vi "Refname to String (Actuator).vi"(1 "Actuator Refname":T1) -> (0 "Refnum Name":string)   [LabVIEW 2015, in "Sprocket.lvlib"]
uses:
  lib/Sprocket.lvlib
  Actuators.ctl
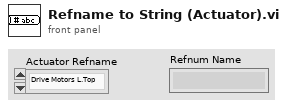
[diagram p1: front panel]
types:
  T1 = typedef "Sprocket.lvlib/Actuators.ctl" = enum16{"Drive Motors L.Top", "Drive Motors R.Top", "Drive Motors L.Bot", "Drive Motors R.Bot", "Collector Motor"}
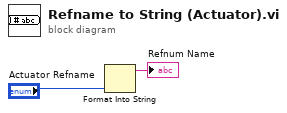
[diagram p0: block diagram]
diagram:
  n1 = Format Into String("Actuator Refname") -> (resulting string=→"Refnum Name":string)  [unwired: 3 in, 1 out]
